vi "[SubVI]ML_Conversion.vi"(2 "Steps":dbl, 3 "Previous LMag":dbl, 4 "Previous RMag":dbl, 5 "Max Mag":dbl, 6 "Array in":dbl[](array[numeric])) -> (0 "Left Torque Command":dbl, 1 "Right Torque Command":dbl)   [LabVIEW 2018]
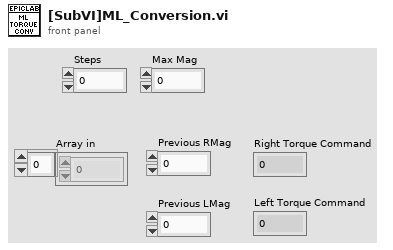
[diagram p1: front panel]
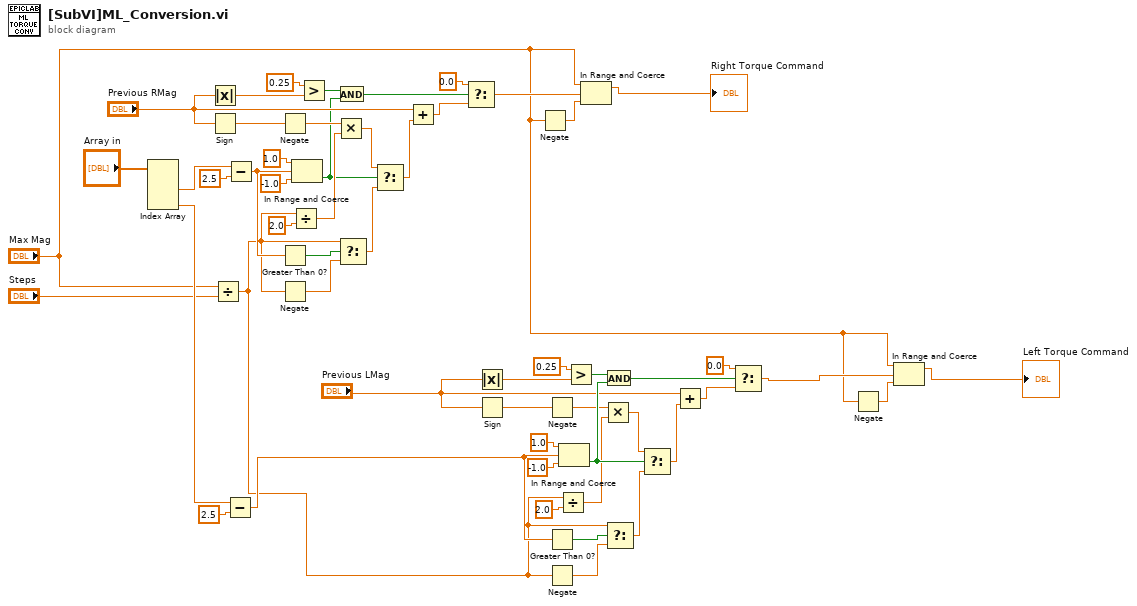
[diagram p0: block diagram]
diagram:
  n1 = Index Array(array="Array in") -> (element #2=w52:dbl, element #4=w54:dbl)  [unwired: 4 in, 2 out]
  n2 = Absolute Value(x="Previous RMag") -> (abs(x)=w48:dbl)
  n3 = Sign(1:"Previous RMag") -> (0:w42:dbl)
  n4 = Divide(x="Max Mag", y="Steps") -> (x/y=w8:dbl)
  n5 = Subtract(x=w54, y=2.5) -> (x-y=w9:dbl)
  n6 = Subtract(x=w52, y=2.5) -> (x-y=w38:dbl)
  n7 = Negate(x=w42) -> (-x=w39:dbl)
  n8 = Greater Than 0?(x=w38) -> (x > 0?=w37:bool)
  n9 = Negate(x=w8) -> (-x=w36:dbl)
  n10 = Divide(x=w8, y=2.0) -> (x/y=w40:dbl)
  n11 = In Range and Coerce(upper limit=1.0, x=w38, lower limit=-1.0) -> (In Range?=w29:bool)  [unwired: 1 out]
  n12 = Greater?(x=0.25, y=w48) -> (0:w30:bool)
  n13 = Multiply(x=w39, y=w40) -> (x*y=w41:dbl)
  n14 = And(x=w30, y=w29) -> (x .and. y?=w31:bool)
  n15 = Select(t=w8, s=w37, f=w36) -> (s? t:f=w35:dbl)
  n16 = Select(t=w41, s=w29, f=w35) -> (s? t:f=w34:dbl)
  n17 = Add(x="Previous RMag", y=w34) -> (x+y=w32:dbl)
  n18 = Select(t=0.0, s=w31, f=w32) -> (s? t:f=w7:dbl)
  n19 = Absolute Value(x="Previous LMag") -> (abs(x)=w11:dbl)
  n20 = Sign(1:"Previous LMag") -> (0:w17:dbl)
  n21 = Negate(x="Max Mag") -> (-x=w6:dbl)
  n22 = Negate(x=w17) -> (-x=w20:dbl)
  n23 = Greater Than 0?(x=w9) -> (x > 0?=w21:bool)
  n24 = Negate(x=w8) -> (-x=w22:dbl)
  n25 = Divide(x=w8, y=2.0) -> (x/y=w19:dbl)
  n26 = In Range and Coerce(upper limit=1.0, x=w9, lower limit=-1.0) -> (In Range?=w28:bool)  [unwired: 1 out]
  n27 = Greater?(x=0.25, y=w11) -> (0:w27:bool)
  n28 = In Range and Coerce(upper limit="Max Mag", x=w7, lower limit=w6) -> (coerced(x)=→"Right Torque Command":dbl)  [unwired: 1 out]
  n29 = Multiply(x=w20, y=w19) -> (x*y=w18:dbl)
  n30 = And(x=w27, y=w28) -> (x .and. y?=w26:bool)
  n31 = Select(t=w8, s=w21, f=w22) -> (s? t:f=w23:dbl)
  n32 = Select(t=w18, s=w28, f=w23) -> (s? t:f=w24:dbl)
  n33 = Add(x="Previous LMag", y=w24) -> (x+y=w25:dbl)
  n34 = Select(t=0.0, s=w26, f=w25) -> (s? t:f=w2:dbl)
  n35 = Negate(x="Max Mag") -> (-x=w4:dbl)
  n36 = In Range and Coerce(upper limit="Max Mag", x=w2, lower limit=w4) -> (coerced(x)=→"Left Torque Command":dbl)  [unwired: 1 out]
